vi "Read Test Stand Class.vi"(8 "error in (no error)":errorcluster, 11 "Init UI Process in":refnum<class "Init UI Process.lvclass">) -> (0 "error out":errorcluster, 2 "Generic Test Stand.lvclass":refnum<class "Generic Test Stand.lvclass">, 3 "Init UI Process out":refnum<class "Init UI Process.lvclass">)   [LabVIEW 2019, in "User Interface Process.lvlib" / "Init UI Process.lvclass"]
uses:
  Init UI Process.lvclass
  Generic Test Stand/Generic Test Stand.lvclass
  Init UI Process.lvclass/Init UI Process.ctl
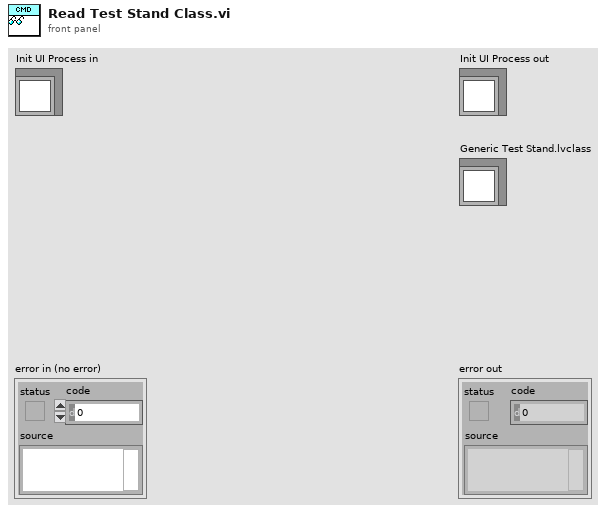
[diagram p1: front panel]
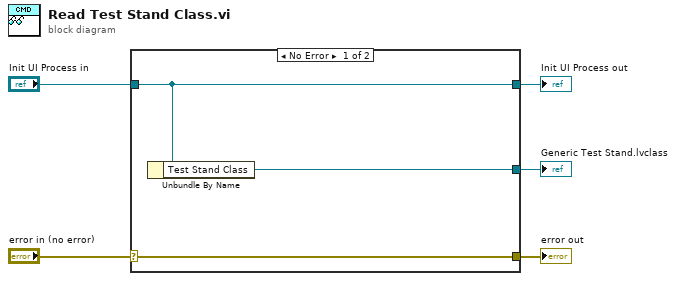
[diagram p0: block diagram]
diagram:
  n1 = case shown="No Error" "error in (no error)" {
    selector: "error in (no error)" -> [w8 w9]
    tunnel: [w8 w9] -> w4
    tunnel: [w7 w10] -> w2
    tunnel: "Init UI Process in" -> [w7 w10]
    tunnel: [w6 _] -> w1
    frame No Error {
      n2 = Unbundle By Name(w7) -> ("Test Stand Class"=w6:refnum<class "Generic Test Stand.lvclass">)
    }
    frame Error {
    }
  }
  "error out" <- w4
  "Init UI Process out" <- w2
  "Generic Test Stand.lvclass" <- w1
